vi "Test MQTT-3.1.3-9.vi"(8 "error in (no error)":errorcluster) -> (0 "error out":errorcluster)   [LabVIEW 2013]
uses:
  source/Control Packets/CONNACK/CONNACK.lvclass
  source/Control Packets/CONNACK/Connect Return Code -- enum.ctl
  source/Server/Connection/TCPConnection.lvclass
  source/Control Packets/CONNECT/CONNECT.lvclass
  source/Control Packets/ControlPacket/ControlPacket.lvclass
  <vilib>/addons/_JKI Toolkits/Caraya/classes/Test/Test.lvclass
  <vilib>/addons/_JKI Toolkits/Caraya/classes/Assert/Assert.lvclass
  source/Control Packets/DISCONNECT/DISCONNECT.lvclass
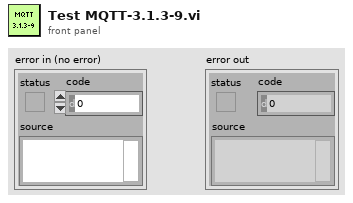
[diagram p1: front panel]
types:
  T1 = enum16{"Standard", "Buffered", "CRLF", "Immediate"}
  T2 = typedef "CONNACK.lvclass/Connect Return Code -- enum.ctl" = enum16{"Connection accepted", "Unacceptable protocol version", "Identifier Rejected", "Server Unavailable", "Bad Username or Password", "Not Authorized"}
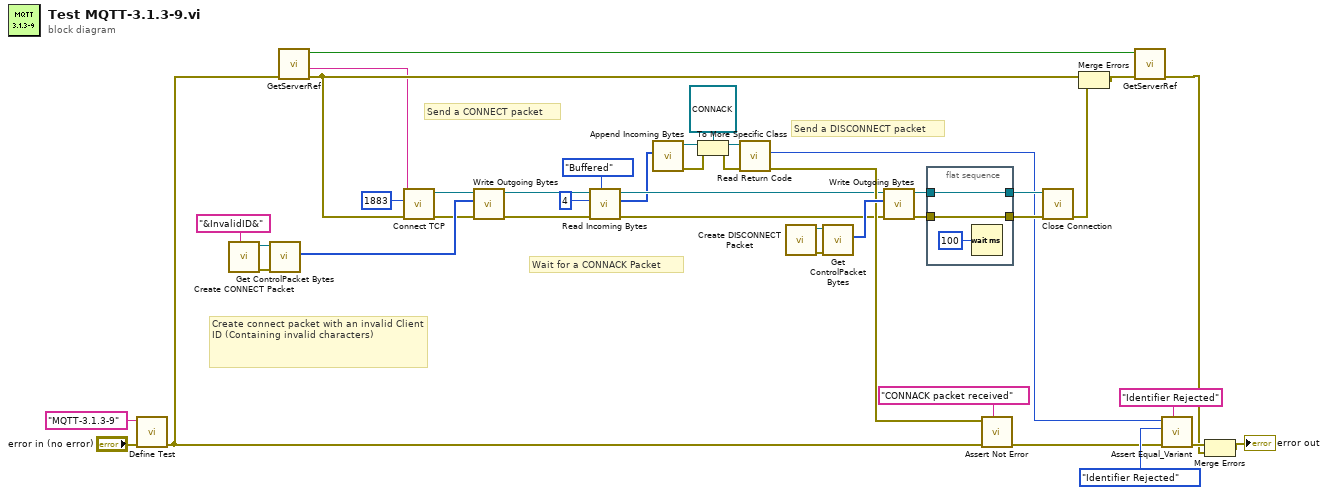
[diagram p0: block diagram]
diagram:
  # "Send a DISCONNECT packet"
  # "Wait for a CONNACK Packet"
  # "Create connect packet with an invalid Client ID (Containing invalid characters)"
  # "Send a CONNECT packet"
  n1 = call <vilib>:"Define Test.vi"("error in (no error)"="error in (no error)", "Label (VI Title)"="MQTT-3.1.3-9") -> ("error out"=w5:errorcluster)  [unwired: 9 in]
  n2 = call "Create CONNECT Packet.vi"("Client ID (empty: generate new)"="&InvalidID&") -> ("error out"=w42:errorcluster, "CONNECT"=w43:refnum<class "CONNECT.lvclass">)  [unwired: 9 in]
  n3 = call "Get ControlPacket Bytes.vi"("error in (no error)"=w42, "ControlPacket"=w43) -> ("Bytes Stream"=w10:u8[])  [unwired: 7 in, 2 out]
  n4 = call "GetServerRef.vi"("error in"=w5) -> ("error out"=w4:errorcluster, "Server address"=w1:string, "Created"=w6:bool)  [unwired: 7 in, 1 out]
  n5 = call "Connect TCP.vi"("error in (no error)"=w4, "remote port (80)"=u16 1883, "address (localhost)"=w1) -> ("error out"=w7:errorcluster, "TCPConnection out"=w8:refnum<class "TCPConnection.lvclass">)  [unwired: 7 in]
  n6 = call "Write Outgoing Bytes.vi"("error in (no error)"=w7, "Bytes"=w10, "TCPConnection in"=w8) -> ("error out"=w16:errorcluster, "TCPConnection out"=w17:refnum<class "TCPConnection.lvclass">)  [unwired: 7 in]
  n7 = call "Read Incoming Bytes.vi"("mode (standard)"=T1."Buffered", "error in (no error)"=w16, "bytes to read (100)"=4 ("bytes to read"), "TCPConnection in"=w17) -> ("error out"=w13:errorcluster, "Bytes"=w12:u8[], "TCPConnection out"=w14:refnum<class "TCPConnection.lvclass">)  [unwired: 4 in, 1 out]
  n8 = call "Append Incoming Bytes.vi"("Incoming Packets"=w12) -> ("error out"=w19:errorcluster, "ControlPacket"=w29:refnum<class "ControlPacket.lvclass">)  [unwired: 7 in, 2 out]
  n9 = To More Specific Class(target class=refnum<class "CONNACK.lvclass"> refnum ("CONNACK.lvclass"), reference=w29, error in=w19) -> (specific class reference=w27:refnum<class "CONNACK.lvclass">, error out=w23:errorcluster)
  n10 = call "Read Return Code.vi"("error in (no error)"=w23, "CONNACK in"=w27) -> ("error out"=w21:errorcluster, "Return Code"=w25:T2)  [unwired: 7 in, 1 out]
  n11 = call "Create DISCONNECT Packet.vi"() -> ("error out"=w35:errorcluster, "DISCONNECT"=w34:refnum<class "DISCONNECT.lvclass">)  [unwired: 10 in]
  n12 = call "Get ControlPacket Bytes.vi"("error in (no error)"=w35, "ControlPacket"=w34) -> ("Bytes Stream"=w33:u8[])  [unwired: 7 in, 2 out]
  n13 = call "Write Outgoing Bytes.vi"("error in (no error)"=w13, "Bytes"=w33, "TCPConnection in"=w14) -> ("error out"=w31:errorcluster, "TCPConnection out"=w32:refnum<class "TCPConnection.lvclass">)  [unwired: 7 in]
  n14 = flat-sequence {
    tunnel: w32 -> [w46]
    tunnel: [w46] -> w30
    tunnel: [w44] -> w26
    tunnel: w31 -> [w44]
    frame #0 {
      n15 = Wait (ms)(milliseconds to wait=u32 100) -> ()  [unwired: 1 out]
    }
  }
  n16 = call <vilib>:"Assert Not Error.vi"("Label"="CONNACK packet received", "error in (no error)"=w5, "Not Error?"=w21) -> ("error out"=w22:errorcluster)  [unwired: 8 in]
  n17 = call-dynamic "Close Connection.vi"("error in (no error)"=w26, "TCPConnection in"=w30) -> ("error out"=w37:errorcluster)  [unwired: 8 in, 1 out]
  n18 = Merge Errors(w4, w37) -> (w3:errorcluster)
  n19 = call "GetServerRef.vi"("error in"=w3, "Destroy (F)"=w6) -> ("error out"=w2:errorcluster)  [unwired: 6 in, 3 out]
  n20 = call <vilib>:"Assert Equal_Variant.vi"("Label"="Identifier Rejected", "error in (no error)"=w22, "Y"=Connect_Return_Code_--_enum."Identifier Rejected" ("Return Code"), "X"=w25) -> ("error out"=w40:errorcluster)  [unwired: 7 in]
  n21 = Merge Errors(w40, w2) -> (→"error out":errorcluster)
